vi "BRig_RT_comm_tcp_write_RTwrite__RunState_Trial_selResult.vi"(7 "input_dataTrial":u16[][](array[numeric]), 10 "iReward_or_iError":bool, 11 "input_dataCurrent":u16[](array[numeric])) -> (2 "output_strCmd":string)   [LabVIEW 2014]
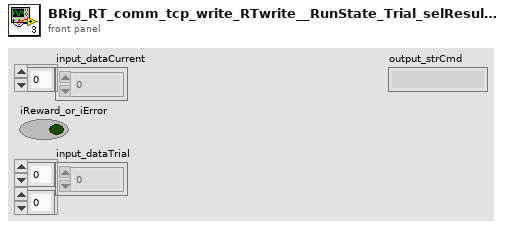
[diagram p1: front panel]
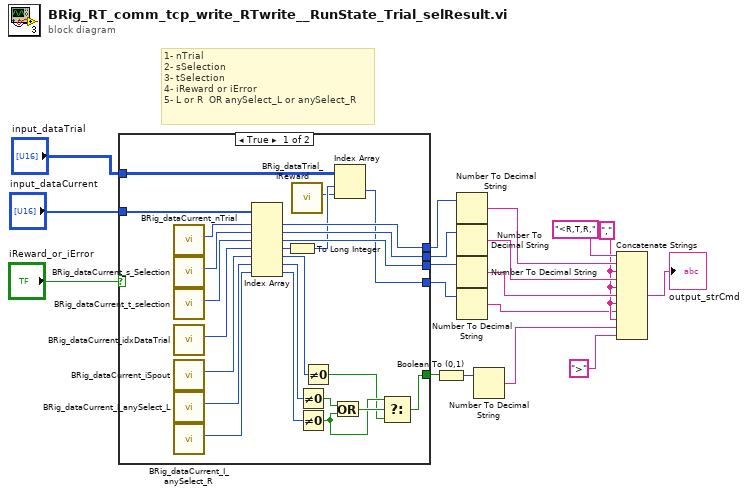
[diagram p0: block diagram]
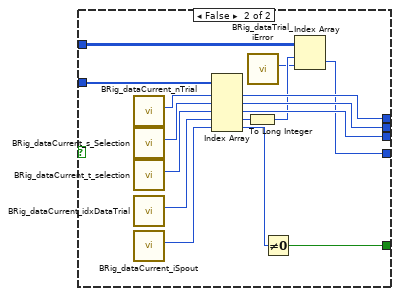
[diagram p2: hidden frame]
diagram:
  w4 = "," ("string")
  # "1- nTrial\n2- sSelection\n3- tSelection\n4- iReward or iError\n5- L or R  OR anySelect_L or anySelect_R"
  n1 = case shown="True" "iReward_or_iError" {
    tunnel: "input_dataCurrent" -> [w41 w57]
    tunnel: [w38 w54] -> w11
    tunnel: [w37 w53] -> w10
    tunnel: [w36 w52] -> w9
    tunnel: "input_dataTrial" -> [w32 w48]
    tunnel: [w30 w47] -> w8
    tunnel: [w19 w44] -> w13
    frame True {
      n2 = call "BRig_dataCurrent_nTrial.vi"() -> ("output_nTrial"=w42:i32)  [unwired: 11 in]
      n3 = call "BRig_dataCurrent_s_Selection.vi"() -> ("output_s_Selection"=w40:i32)  [unwired: 11 in]
      n4 = call "BRig_dataCurrent_t_selection.vi"() -> ("output_t_selection"=w39:i32)  [unwired: 11 in]
      n5 = call "BRig_dataCurrent_idxDataTrial.vi"() -> ("output_idxDataTrial"=w35:i32)  [unwired: 11 in]
      n6 = call "BRig_dataCurrent_iSpout.vi"() -> ("output_iSpout"=w29:i32)  [unwired: 11 in]
      n7 = call "BRig_dataCurrent_I_anySelect_L.vi"() -> ("output_IanySelect_L"=w28:i32)  [unwired: 11 in]
      n8 = call "BRig_dataCurrent_I_anySelect_R.vi"() -> ("output_IanySelect_R"=w27:i32)  [unwired: 11 in]
      n9 = Index Array(array=w41, index #1=w42, index #2=w40, index #3=w39, index #4=w35, index #5=w29, index #6=w28, index #7=w27) -> (element #1=w38:u16, element #2=w37:u16, element #3=w36:u16, element #4=w34:u16, element #5=w21:u16, element #6=w26:u16, element #7=w25:u16)
      n10 = To Long Integer(number=w34) -> (32bit integer=w33:i32)
      n11 = call "BRig_dataTrial_iReward.vi"() -> ("output_iReward"=w31:i32)  [unwired: 11 in]
      n12 = Not Equal To 0?(x=w26) -> (x != 0?=w24:bool)
      n13 = Not Equal To 0?(x=w25) -> (x != 0?=w22:bool)
      n14 = Not Equal To 0?(x=w21) -> (x != 0?=w20:bool)
      n15 = Or(x=w24, y=w22) -> (x .or. y?=w23:bool)
      n16 = Index Array(array=w32, index (row)=w33, index (col)=w31) -> (element=w30:u16)
      n17 = Select(t=w22, s=w23, f=w20) -> (s? t:f=w19:bool)
    }
    frame False {
      n18 = call "BRig_dataCurrent_nTrial.vi"() -> ("output_nTrial"=w58:i32)  [unwired: 11 in]
      n19 = call "BRig_dataCurrent_s_Selection.vi"() -> ("output_s_Selection"=w56:i32)  [unwired: 11 in]
      n20 = call "BRig_dataCurrent_t_selection.vi"() -> ("output_t_selection"=w55:i32)  [unwired: 11 in]
      n21 = call "BRig_dataCurrent_idxDataTrial.vi"() -> ("output_idxDataTrial"=w51:i32)  [unwired: 11 in]
      n22 = call "BRig_dataCurrent_iSpout.vi"() -> ("output_iSpout"=w46:i32)  [unwired: 11 in]
      n23 = Index Array(array=w57, index #1=w58, index #2=w56, index #3=w55, index #4=w51, index #5=w46) -> (element #1=w54:u16, element #2=w53:u16, element #3=w52:u16, element #4=w50:u16, element #5=w45:u16)
      n24 = To Long Integer(number=w50) -> (32bit integer=w49:i32)
      n25 = call "BRig_dataTrial_iError.vi"() -> ("output_iError"=w43:i32)  [unwired: 11 in]
      n26 = Not Equal To 0?(x=w45) -> (x != 0?=w44:bool)
      n27 = Index Array(array=w48, index (row)=w49, index (col)=w43) -> (element=w47:u16)
    }
  }
  n28 = Boolean To (0,1)(Boolean=w13) -> (0, 1=w12:i16)
  n29 = Number To Decimal String(number=w11) -> (decimal integer string=w7:string)  [unwired: 1 in]
  n30 = Number To Decimal String(number=w10) -> (decimal integer string=w6:string)  [unwired: 1 in]
  n31 = Number To Decimal String(number=w9) -> (decimal integer string=w5:string)  [unwired: 1 in]
  n32 = Number To Decimal String(number=w8) -> (decimal integer string=w3:string)  [unwired: 1 in]
  n33 = Number To Decimal String(number=w12) -> (decimal integer string=w2:string)  [unwired: 1 in]
  n34 = Concatenate Strings("<R,T,R," ("string"), w7, w4, w6, w4, w5, w4, w3, w4, w2, ">" ("string")) -> (→"output_strCmd":string)
